vi "rszvl_core_global.vi"() -> ()   [LabVIEW 2014] (continued)
"*WAI"=FALSE}, "Check Status Callback"=""}, {"Level"=2, "Descriptive Name"="File Decimal Separator", "Class Only"=FALSE, "Data Type"=0, "Access"=2, "Identifier"="RSZVL_ATTR_FILE_DEC_SEPARATOR", "Range Table"="rszvl_rngFileDecSeparator", "Command"="FORM:DEXP:DSEP", "Read Callback"="", "Write Callback"="", "Range Callback"="", "Check Callback"="", "Rngtable Callback"="", "Coerce Callback"="", "User Callback"="", "Supported Models"="", "Instrument Options"="", "Repeated Capabilities"="", "Restricted Repeated Capabilities"="", "Help"="This attribute defines which decimal separator (decimal point or comma) is to be used for outputting measurement data to the file in ASCII format.\n\nAvailable Repeated Capabilities:\nNone\n\nRemote-control command(s):\nFORMat:DEXPort:DSEParator POINt|COMMa", "Flags"={"OPC Wait"=FALSE, "Dont check status"=FALSE, "*WAI"=FALSE}, "Check Status Callback"=""}, {"Level"=2, "Descriptive Name"="Manager", "Class Only"=TRUE, "Data Type"=0, "Access"=0, "Identifier"="", "Range Table"="", "Command"="", "Read Callback"="", "Write Callback"="", "Range Callback"="", "Check Callback"="", "Rngtable Callback"="", "Coerce Callback"="", "User Callback"="", "Supported Models"="", "Instrument Options"="", "Repeated Capabilities"="", "Restricted Repeated Capabilities"="", "Help"="File management attributes.\n\n(1) File Manager Edit Path:\nThis attribute changes the current directory.\nIn addition to the path name, the indication of the directory may contain the drive name. The path name complies with the DOS conventions.\n\n(2) File Manager Delete:\n\n\n(3) File Manager Make Directory:\nThis attribute creates a new directory. The file name includes indication of the path and may also include the drive name. The path name complies with DOS conventions.\n\n(4) File Manager Edit Path Device:\nThis attribute changes to the drive indicated. The drive may be the internal hard disk D: or the floppy disk drive A:.\n\n(5) File Manager Delete Directory:\nThis attribute deletes the indicated directory. The directory name includes indication of the path and may also include the drive name. The path name complies with DOS conventions.", "Flags"={"OPC Wait"=FALSE, "Dont check status"=FALSE, "*WAI"=FALSE}, "Check Status Callback"=""}, {"Level"=3, "Descriptive Name"="File Manager Edit Path", "Class Only"=FALSE, "Data Type"=2, "Access"=2, "Identifier"="RSZVL_ATTR_FILE_MANAGER_EDIT_PATH", "Range Table"="", "Command"="MMEM:CDIR", "Read Callback"="rszvl_quotedString_ReadCallback.vi", "Write Callback"="rszvl_quotedString_WriteCallback.vi", "Range Callback"="", "Check Callback"="", "Rngtable Callback"="", "Coerce Callback"="", "User Callback"="", "Supported Models"="", "Instrument Options"="", "Repeated Capabilities"="", "Restricted Repeated Capabilities"="", "Help"="This attribute changes the current directory.\nIn addition to the path name, the indication of the directory may contain the drive name. The path name complies with the DOS conventions.\n\nAvailable Repeated Capabilities:\nNone\n\nRemote-control command(s):\nMMEMory:CDIRectory", "Flags"={"OPC Wait"=FALSE, "Dont check status"=FALSE, "*WAI"=FALSE}, "Check Status Callback"=""}, {"Level"=3, "Descriptive Name"="File Manager Delete", "Class Only"=FALSE, "Data Type"=2, "Access"=1, "Identifier"="RSZVL_ATTR_FILE_MANAGER_DELETE", "Range Table"="", "Command"="MMEM:DEL", "Read Callback"="", "Write Callback"="", "Range Callback"="", "Check Callback"="", "Rngtable Callback"="", "Coerce Callback"="", "User Callback"="", "Supported Models"="", "Instrument Options"="", "Repeated Capabilities"="", "Restricted Repeated Capabilities"="", "Help"="\n\nAvailable Repeated Capabilities:\nNone\n\nRemote-control command(s):\nMMEMory:DELete", "Flags"={"OPC Wait"=FALSE, "Dont check status"=FALSE, "*WAI"=FALSE}, "Check Status Callback"=""}, {"Level"=3, "Descriptive Name"="File Manager Make Directory", "Class Only"=FALSE, "Data Type"=2, "Access"=2, "Identifier"="RSZVL_ATTR_FILE_MANAGER_MAKE_DIR", "Range Table"="", "Command"="MMEM:MDIR", "Read Callback"="", "Write Callback"="", "Range Callback"="", "Check Callback"="", "Rngtable Callback"="", "Coerce Callback"="", "User Callback"="", "Supported Models"="", "Instrument Options"="", "Repeated Capabilities"="", "Restricted Repeated Capabilities"="", "Help"="This attribute creates a new directory. The file name includes indication of the path and may also include the drive name. The path name complies with DOS conventions.\n\nAvailable Repeated Capabilities:\nNone\n\nRemote-control command(s):\nMMEMory:MDIRectory", "Flags"={"OPC Wait"=FALSE, "Dont check status"=FALSE, "*WAI"=FALSE}, "Check Status Callback"=""}, {"Level"=3, "Descriptive Name"="File Manager Edit Path Device", "Class Only"=FALSE, "Data Type"=2, "Access"=2, "Identifier"="RSZVL_ATTR_FILE_MANAGER_EDIT_PATH_DEVICE", "Range Table"="", "Command"="MMEM:MSIS", "Read Callback"="rszvl_quotedString_ReadCallback.vi", "Write Callback"="rszvl_quotedString_WriteCallback.vi", "Range Callback"="", "Check Callback"="", "Rngtable Callback"="", "Coerce Callback"="", "User Callback"="", "Supported Models"="", "Instrument Options"="", "Repeated Capabilities"="", "Restricted Repeated Capabilities"="", "Help"="This attribute changes to the drive indicated. The drive may be the internal hard disk D: or the floppy disk drive A:.\n\nAvailable Repeated Capabilities:\nNone\n\nRemote-control command(s):\nMMEMory:MSIS", "Flags"={"OPC Wait"=FALSE, "Dont check status"=FALSE, "*WAI"=FALSE}, "Check Status Callback"=""}, {"Level"=3, "Descriptive Name"="File Manager Delete Directory", "Class Only"=FALSE, "Data Type"=2, "Access"=2, "Identifier"="RSZVL_ATTR_FILE_MANAGER_DELETE_DIR", "Range Table"="", "Command"="MMEM:RDIR", "Read Callback"="", "Write Callback"="", "Range Callback"="", "Check Callback"="", "Rngtable Callback"="", "Coerce Callback"="", "User Callback"="", "Supported Models"="", "Instrument Options"="", "Repeated Capabilities"="", "Restricted Repeated Capabilities"="", "Help"="This attribute deletes the indicated directory. The directory name includes indication of the path and may also include the drive name. The path name complies with DOS conventions.\n\nAvailable Repeated Capabilities:\nNone\n\nRemote-control command(s):\nMMEMory:RDIRectory", "Flags"={"OPC Wait"=FALSE, "Dont check status"=FALSE, "*WAI"=FALSE}, "Check Status Callback"=""}, {"Level"=2, "Descriptive Name"="Save Recall", "Class Only"=TRUE, "Data Type"=0, "Access"=0, "Identifier"="", "Range Table"="", "Command"="", "Read Callback"="", "Write Callback"="", "Range Callback"="", "Check Callback"="", "Rngtable Callback"="", "Coerce Callback"="", "User Callback"="", "Supported Models"="", "Instrument Options"="", "Repeated Capabilities"="", "Restricted Repeated Capabilities"="", "Help"="Configuration of stored setups.\n\n(1) File Items to Save Recall Select Source Cal Data:\nThis attribute adds the tracking generator calibration data to the list of device settings to be stored/loaded.\n\n(2) File Items to Save Recall Select All Transducers:\nThis attribute includes all transducer factors and sets in the list of data subsets of a device setting to be stored/loaded.\n\n(3) File Items to Save Recall Select HW Settings:\nThis attribute includes the hardware settings in the list of data subsets of a device setting to be stored/loaded. The hardware settings include:\n- current configuration of general device parameters (general setup)\n- current setting of the measurement hardware including markers\n- activated limit lines:\nA data set may include 8 limit lines at maximum. This number includes the activated limit lines and, if available, the de-activated limit lines last used. Therefore the combination of the non-activated restored limit lines depends on the sequence of use with the command MMEM:LOAD.\n- user-defined color setting\n- configuration for the hardcopy output\n- Tracking generator settings (only in conjunction with option External Generator Control B10)\n- Correction data for source calibration (only in conjunction with option External Generator Control B10)\n\n(4) File Items to Save Recall Select Trace:\nThis attribute adds the active traces to the list of data subsets of a save/recall device setting. Active traces are all traces whose state is not blank.\n\n(5) File Items to Save Recall Select Lines:\nThis attribute adds all limit lines (activated and de-activated) to the list of device settings to be\nstored/loaded.\n\n(6) File Items to Save Recall All:\nThis command includes all data subsets in the list device settings to be stored/loaded.\n\n(7) File Items to Save Recall None:\nThis attribute deletes all data subsets from the list of device settings to be stored/loaded.\n\n(8) File Items to Save Recall Default:\nThis attribute sets the default list of device settings to be stored/loaded.The latter includes:\n- current configuration of general device parameters (general setup)\n- current setting of the measurement hardware including markers\n- activated limit lines\n- user-defined color setting\n- configuration for the hardcopy output\n- Tracking generator settings (only in conjunction with option External Generator Control B10)\n- Correction data for source calibration (only in conjunction with option External Generator Control B10)\nTrace data and non-used limit lines are not included.", "Flags"={"OPC Wait"=FALSE, "Dont check status"=FALSE, "*WAI"=FALSE}, "Check Status Callback"=""}, {"Level"=3, "Descriptive Name"="File Items to Save Recall Select Source Cal Data", "Class Only"=FALSE, "Data Type"=3, "Access"=2, "Identifier"="RSZVL_ATTR_FILE_ITEMS_SAVE_RECAL_SEL_SOURCE_CAL_DATA", "Range Table"="", "Command"="MMEM:SEL:SCD", "Read Callback"="", "Write Callback"="", "Range Callback"="", "Check Callback"="", "Rngtable Callback"="", "Coerce Callback"="", "User Callback"="", "Supported Models"="", "Instrument Options"="", "Repeated Capabilities"="", "Restricted Repeated Capabilities"="", "Help"="This attribute adds the tracking generator calibration data to the list of device settings to be stored/loaded.\n\nAvailable Repeated Capabilities:\nNone\n\nRemote-control command(s):\nMMEMory:SELect[:ITEM]:SCData ON | OFF", "Flags"={"OPC Wait"=FALSE, "Dont check status"=FALSE, "*WAI"=FALSE}, "Check Status Callback"=""}, {"Level"=3, "Descriptive Name"="File Items to Save Recall Select All Transducers", "Class Only"=FALSE, "Data Type"=3, "Access"=2, "Identifier"="RSZVL_ATTR_FILE_ITEMS_SAVE_RECAL_SEL_TRAN", "Range Table"="", "Command"="MMEM:SEL:TRAN:ALL", "Read Callback"="", "Write Callback"="", "Range Callback"="", "Check Callback"="", "Rngtable Callback"="", "Coerce Callback"="", "User Callback"="", "Supported Models"="", "Instrument Options"="", "Repeated Capabilities"="", "Restricted Repeated Capabilities"="", "Help"="This attribute includes all transducer factors and sets in the list of data subsets of a device setting to be stored/loaded.\n\nAvailable Repeated Capabilities:\nNone\n\nRemote-control command(s):\nMMEMory:SELect[:ITEM]:TRANsducer:ALL ON | OFF", "Flags"={"OPC Wait"=FALSE, "Dont check status"=FALSE, "*WAI"=FALSE}, "Check Status Callback"=""}, {"Level"=3, "Descriptive Name"="File Items to Save Recall Select HW Settings", "Class Only"=FALSE, "Data Type"=3, "Access"=2, "Identifier"="RSZVL_ATTR_FILE_ITEMS_SAVE_RECAL_SEL_HWSETTINGS", "Range Table"="", "Command"="MMEM:SEL:HWS", "Read Callback"="", "Write Callback"="", "Range Callback"="", "Check Callback"="", "Rngtable Callback"="", "Coerce Callback"="", "User Callback"="", "Supported Models"="", "Instrument Options"="", "Repeated Capabilities"="", "Restricted Repeated Capabilities"="", "Help"="This attribute includes the hardware settings in the list of data subsets of a device setting to be stored/loaded. The hardware settings include:\n- current configuration of general device parameters (general setup)\n- current setting of the measurement hardware including markers\n- activated limit lines:\nA data set may include 8 limit lines at maximum. This number includes the activated limit lines and, if available, the de-activated limit lines last used. Therefore the combination of the non-activated restored limit lines depends on the sequence of use with the command MMEM:LOAD.\n- user-defined color setting\n- configuration for the hardcopy output\n- Tracking generator settings (only in conjunction with option External Generator Control B10)\n- Correction data for source calibration (only in conjunction with option External Generator Control B10)\n\nAvailable Repeated Capabilities:\nNone\n\nRemote-control command(s):\nMMEMory:SELect[:ITEM]:HWSettings ON|OFF", "Flags"={"OPC Wait"=FALSE, "Dont check status"=FALSE, "*WAI"=FALSE}, "Check Status Callback"=""}, {"Level"=3, "Descriptive Name"="File Items to Save Recall Select Trace", "Class Only"=FALSE, "Data Type"=3, "Access"=2, "Identifier"="RSZVL_ATTR_FILE_ITEMS_SAVE_RECAL_SEL_TRAC", "Range Table"="", "Command"="MMEM:SEL:TRAC", "Read Callback"="", "Write Callback"="", "Range Callback"="", "Check Callback"="", "Rngtable Callback"="", "Coerce Callback"="", "User Callback"="", "Supported Models"="", "Instrument Options"="", "Repeated Capabilities"="", "Restricted Repeated Capabilities"="", "Help"="This attribute adds the active traces to the list of data subsets of a save/recall device setting. Active traces are all traces whose state is not blank.\n\nAvailable Repeated Capabilities:\nNone\n\nRemote-control command(s):\nMMEMory:SELect[:ITEM]:TRACe[:ACTive] ON|OFF", "Flags"={"OPC Wait"=FALSE, "Dont check status"=FALSE, "*WAI"=FALSE}, "Check Status Callback"=""}, {"Level"=3, "Descriptive Name"="File Items to Save Recall Select Lines", "Class Only"=FALSE, "Data Type"=3, "Access"=2, "Identifier"="RSZVL_ATTR_FILE_ITEMS_SAVE_RECAL_SEL_LINE", "Range Table"="", "Command"="MMEM:SEL:LIN:ALL", "Read Callback"="", "Write Callback"="", "Range Callback"="", "Check Callback"="", "Rngtable Callback"="", "Coerce Callback"="", "User Callback"="", "Supported Models"="", "Instrument Options"="", "Repeated Capabilities"="", "Restricted Repeated Capabilities"="", "Help"="This attribute adds all limit lines (activated and de-activated) to the list of device settings to be\nstored/loaded.\n\nAvailable Repeated Capabilities:\nNone\n\nRemote-control command(s):\nMMEMory:SELect[:ITEM]:LINes:ALL ON|OFF", "Flags"={"OPC Wait"=FALSE, "Dont check status"=FALSE, "*WAI"=FALSE}, "Check Status Callback"=""}, {"Level"=3, "Descriptive Name"="File Items to Save Recall All", "Class Only"=FALSE, "Data Type"=4, "Access"=1, "Identifier"="RSZVL_ATTR_FILE_ITEMS_SAVE_RECAL_ALL", "Range Table"="", "Command"="MMEM:SEL:ALL", "Read Callback"="", "Write Callback"="", "Range Callback"="", "Check Callback"="", "Rngtable Callback"="", "Coerce Callback"="", "User Callback"="", "Supported Models"="", "Instrument Options"="", "Repeated Capabilities"="", "Restricted Repeated Capabilities"="", "Help"="This command includes all data subsets in the list device settings to be stored/loaded.\n\nAvailable Repeated Capabilities:\nNone\n\nRemote-control command(s):\nMMEMory:SELect[:ITEM]:ALL", "Flags"={"OPC Wait"=FALSE, "Dont check status"=FALSE, "*WAI"=FALSE}, "Check Status Callback"=""}, {"Level"=3, "Descriptive Name"="File Items to Save Recall None", "Class Only"=FALSE, "Data Type"=4, "Access"=1, "Identifier"="RSZVL_ATTR_FILE_ITEMS_SAVE_RECAL_NONE", "Range Table"="", "Command"="MMEM:SEL:NONE", "Read Callback"="", "Write Callback"="", "Range Callback"="", "Check Callback"="", "Rngtable Callback"="", "Coerce Callback"="", "User Callback"="", "Supported Models"="", "Instrument Options"="", "Repeated Capabilities"="", "Restricted Repeated Capabilities"="", "Help"="This attribute deletes all data subsets from the list of device settings to be stored/loaded.\n\nAvailable Repeated Capabilities:\nNone\n\nRemote-control command(s):\nMMEMory:SELect[:ITEM]:NONE", "Flags"={"OPC Wait"=FALSE, "Dont check status"=FALSE, "*WAI"=FALSE}, "Check Status Callback"=""}, {"Level"=3, "Descriptive Name"="File Items to Save Recall Default", "Class Only"=FALSE, "Data Type"=4, "Access"=1, "Identifier"="RSZVL_ATTR_FILE_ITEMS_SAVE_RECAL_DEFAULT", "Range Table"="", "Command"="MMEM:SEL:DEF", "Read Callback"="", "Write Callback"="", "Range Callback"="", "Check Callback"="", "Rngtable Callback"="", "Coerce Callback"="", "User Callback"="", "Supported Models"="", "Instrument Options"="", "Repeated Capabilities"="", "Restricted Repeated Capabilities"="", "Help"="This attribute sets the default list of device settings to be stored/loaded.The latter includes:\n- current configuration of general device parameters (general setup)\n- current setting of the measurement hardware including markers\n- activated limit lines\n- user-defined color setting\n- configuration for the hardcopy output\n- Tracking generator settings (only in conjunction with option External Generator Control B10)\n- Correction data for source calibration (only in conjunction with option External Generator Control B10)\nTrace data and non-used limit lines are not included.\n\nAvailable Repeated Capabilities:\nNone\n\nRemote-control command(s):\nMMEMory:SELect[:ITEM]:DEFault", "Flags"={"OPC Wait"=FALSE, "Dont check status"=FALSE, "*WAI"=FALSE}, "Check Status Callback"=""}, {"Level"=1, "Descriptive Name"="Hard Copy", "Class Only"=TRUE, "Data Type"=0, "Access"=0, "Identifier"="", "Range Table"="", "Command"="", "Read Callback"="", "Write Callback"="", "Range Callback"="", "Check Callback"="", "Rngtable Callback"="", "Coerce Callback"="", "User Callback"="", "Supported Models"="", "Instrument Options"="", "Repeated Capabilities"="", "Restricted Repeated Capabilities"="", "Help"="(1) Hcopy Abort:\nThis attribute aborts a running hardcopy output.\n\n(2) Hcopy Color Default:\nThis attribute resets the colors for a hardcopy to the selected default settings. DEFault1(SCREEN COLORS, but background white), DEFault2 (OPTIMIZED COLOR SET) and DEFault3 (USER DEFINED). The numeric suffix in CMAP is not significant.\n\n(3) Hcopy Color:\nThis attribute selects between color and monochrome hardcopy of the screen.\n\n(4) Hcopy Print:\nThis attribute starts a hardcopy output. The numeric suffix selects which printer configuration (1 or 2) is to be used for the hardcopy output. If there is no suffix, configuration 1 is automatically selected.\n\n(5) Hcopy Print Next:\nThis attribute starts a hardcopy output. If the output is printed to a file (see HCOPy:DESTination<1|2>), the file name used in the last saving process is automatically counted up to the next unused name.\n\n(6) Hcopy Device Destination:\nThis attribute selects the printer output medium (Disk, Printer or Clipboard) associated with configuration 1 or 2.\n\n(7) Hcopy Color Predefined:\nThis attribute defines the color table in USER DEFINED COLORS using predefined color values. To each numeric suffix of CMAP is assigned one or several picture elements which can be modified by varying the corresponding color setting.\n\n(8) Hcopy Device Language Output Format:\nThis attribute determines the data format of the printout. More info in manual.\n\n(9) Hcopy Print Screen:\nThis attribute selects the complete screen to be output.\n\n(10) Hcopy Comment Screen:\nThis attribute defines the comment text for printout, with a maximum of 100 characters; line feed by means of character @).\n\n(11) Hcopy Print Trace:\nThis attribute selects the output of the currently displayed trace.\n\n(12) Hcopy Device Orientation:\n\n\n(13) Hcopy File Name:\nThis attribute defines a destination file for the printout started with the command HCOPy:IMMediate. In this case the printer output must be routed to destination FILE using the attribute RSZVL_ATTR_HCOPY_DEVICE_DESTINATION with MMEM\nThe file name includes indication of the path and may also include the drive name. The file name and path information comply with DOS conventions.\n\n(14) Hardcopy Select Printer:\nThis attribute selects one of the printers configured under Windows NT including the associated output destination.\n\nThe specified printer name must be a string as returned by the commands\nSYSTem:COMMunicate :PRINter:ENUMerate:FIRSt? or\nSYSTem:COMMunicate :PRINter:ENUMerate:NEXT?\n\n(15) Hardcopy Get Next Printer:\nThis attribute queries the name of the next printer installed under Windows NT.\nThe names of other printers can then be queried with NEXT?. After all available printer names have been output, an empty string enclosed by quotation marks is output for the next query. Further queries are answered by a Query Error.\n\n(16) Hardcopy Get First Printer:\nThis attribute queries the name of the first printer (in the list of printers) available under Windows NT.", "Flags"={"OPC Wait"=FALSE, "Dont check status"=FALSE, "*WAI"=FALSE}, "Check Status Callback"=""}, {"Level"=2, "Descriptive Name"="Hcopy Abort", "Class Only"=FALSE, "Data Type"=4, "Access"=1, "Identifier"="RSZVL_ATTR_HCOPY_ABORT", "Range Table"="", "Command"="HCOP:ABOR", "Read Callback"="", "Write Callback"="", "Range Callback"="", "Check Callback"="", "Rngtable Callback"="", "Coerce Callback"="", "User Callback"="", "Supported Models"="", "Instrument Options"="", "Repeated Capabilities"="", "Restricted Repeated Capabilities"="", "Help"="This attribute aborts a running hardcopy output.\n\nAvailable Repeated Capabilities:\nNone\n\nRemote-control command(s):\nHCOPy:ABORt", "Flags"={"OPC Wait"=FALSE, "Dont check status"=FALSE, "*WAI"=FALSE}, "Check Status Callback"=""}, {"Level"=2, "Descriptive Name"="Hcopy Color Default", "Class Only"=FALSE, "Data Type"=4, "Access"=1, "Identifier"="RSZVL_ATTR_HCOPY_COLOR_DEF", "Range Table"="", "Command"="HCOP:CMAP:DEF{Default}", "Read Callback"="", "Write Callback"="", "Range Callback"="", "Check Callback"="", "Rngtable Callback"="", "Coerce Callback"="", "User Callback"="", "Supported Models"="", "Instrument Options"="", "Repeated Capabilities"="", "Restricted Repeated Capabilities"="", "Help"="This attribute resets the colors for a hardcopy to the selected default settings. DEFault1(SCREEN COLORS, but background white), DEFault2 (OPTIMIZED COLOR SET) and DEFault3 (USER DEFINED). The numeric suffix in CMAP is not significant.\n\nAvailable Repeated Capabilities:\nDefault: DEF1,DEF2,DEF3\r\n\nRemote-control command(s):\nHCOPy:CMAP<1 to 27>:DEFault1|2|3", "Flags"={"OPC Wait"=FALSE, "Dont check status"=FALSE, "*WAI"=FALSE}, "Check Status Callback"=""}, {"Level"=2, "Descriptive Name"="Hcopy Color", "Class Only"=FALSE, "Data Type"=3, "Access"=2, "Identifier"="RSZVL_ATTR_HCOPY_COLOR", "Range Table"="", "Command"="HCOP:DEV:COL", "Read Callback"="", "Write Callback"="", "Range Callback"="", "Check Callback"="", "Rngtable Callback"="", "Coerce Callback"="", "User Callback"="", "Supported Models"="", "Instrument Options"="", "Repeated Capabilities"="", "Restricted Repeated Capabilities"="", "Help"="This attribute selects between color and monochrome hardcopy of the screen.\n\nAvailable Repeated Capabilities:\nNone\n\nRemote-control command(s):\nHCOPy:DEVice:COLor ON|OFF", "Flags"={"OPC Wait"=FALSE, "Dont check status"=FALSE, "*WAI"=FALSE}, "Check Status Callback"=""}, {"Level"=2, "Descriptive Name"="Hcopy Print", "Class Only"=FALSE, "Data Type"=4, "Access"=1, "Identifier"="RSZVL_ATTR_HCOPY_PRINT", "Range Table"="", "Command"="HCOP:IMM{Destination}", "Read Callback"="", "Write Callback"="", "Range Callback"="", "Check Callback"="", "Rngtable Callback"="", "Coerce Callback"="", "User Callback"="", "Supported Models"="", "Instrument Options"="", "Repeated Capabilities"="", "Restricted Repeated Capabilities"="", "Help"="This attribute starts a hardcopy output. The numeric suffix selects which printer configuration (1 or 2) is to be used for the hardcopy output. If there is no suffix, configuration 1 is automatically selected.\n\nAvailable Repeated Capabilities:\nDestination: DE1,DE2\r\n\nRemote-control command(s):\nHCOPy[:IMMediate<1|2>]", "Flags"={"OPC Wait"=FALSE, "Dont check status"=FALSE, "*WAI"=FALSE}, "Check Status Callback"=""}, {"Level"=2, "Descriptive Name"="Hcopy Print Next", "Class Only"=FALSE, "Data Type"=4, "Access"=1, "Identifier"="RSZVL_ATTR_HCOPY_PRINT_NEXT", "Range Table"="", "Command"="HCOP:IMM{Destination}:NEXT", "Read Callback"="", "Write Callback"="", "Range Callback"="", "Check Callback"="", "Rngtable Callback"="", "Coerce Callback"="", "User Callback"="", "Supported Models"="", "Instrument Options"="", "Repeated Capabilities"="", "Restricted Repeated Capabilities"="", "Help"="This attribute starts a hardcopy output. If the output is printed to a file (see HCOPy:DESTination<1|2>), the file name used in the last saving process is automatically counted up to the next unused name.\n\nAvailable Repeated Capabilities:\nDestination: DE1,DE2\r\n\nRemote-control command(s):\nHCOPy[:IMMediate<config>]:NEXT", "Flags"={"OPC Wait"=FALSE, "Dont check status"=FALSE, "*WAI"=FALSE}, "Check Status Callback"=""}, {"Level"=2, "Descriptive Name"="Hcopy Device Destination", "Class Only"=FALSE, "Data Type"=0, "Access"=2, "Identifier"="RSZVL_ATTR_HCOPY_DEVICE_DESTINATION", "Range Table"="rszvl_rngHcopyDevice", "Command"="HCOP:DEST{Destination}", "Read Callback"="", "Write Callback"="", "Range Callback"="", "Check Callback"="", "Rngtable Callback"="", "Coerce Callback"="", "User Callback"="", "Supported Models"="", "Instrument Options"="", "Repeated Capabilities"="", "Restricted Repeated Capabilities"="", "Help"="This attribute selects the printer output medium (Disk, Printer or Clipboard) associated with configuration 1 or 2.\n\nAvailable Repeated Capabilities:\nDestination: DE1,DE2\r\n\nRemote-control command(s):\nHCOPy:DESTination<1|2>", "Flags"={"OPC Wait"=FALSE, "Dont check status"=FALSE, "*WAI"=FALSE}, "Check Status Callback"=""}, {"Level"=2, "Descriptive Name"="Hcopy Color Predefined", "Class Only"=FALSE, "Data Type"=0, "Access"=1, "Identifier"="RSZVL_ATTR_HCOPY_COLOR_PREDEFINED", "Range Table"="rszvl_rngDISPConfPreDefColour", "Command"="HCOP:CMAP{CMAP}:PDEF", "Read Callback"="", "Write Callback"="", "Range Callback"="", "Check Callback"="", "Rngtable Callback"="", "Coerce Callback"="", "User Callback"="", "Supported Models"="", "Instrument Options"="", "Repeated Capabilities"="", "Restricted Repeated Capabilities"="", "Help"="This attribute defines the color table in USER DEFINED COLORS using predefined color values. To each numeric suffix of CMAP is assigned one or several picture elements which can be modified by varying the corresponding color setting.\n\nAvailable Repeated Capabilities:\nCMAP: CM1,CM2,CM3,CM4,CM5,CM6,CM7,CM8,CM9,CM10,CM11,CM12,CM13,CM14,CM15,CM16,CM17,CM18,CM19,CM20,CM21,CM22,CM23,CM24,CM25,CM26,CM27\r\n\nRemote-control command(s):\nHCOPy:CMAP<1 to 26>:PDEFined BLACk | BLUE | BROWn | GREen | CYAN | RED | MAGenta | YELLow | WHITe | DGRAy | LGRAy | LBLUe | LGREen | LCYan | LRED | LMAGenta", "Flags"={"OPC Wait"=FALSE, "Dont check status"=FALSE, "*WAI"=FALSE}, "Check Status Callback"=""}, {"Level"=2, "Descriptive Name"="Hcopy Device Language Output Format", "Class Only"=FALSE, "Data Type"=0, "Access"=2, "Identifier"="RSZVL_ATTR_HCOPY_DEVICE_LANG_OUT_FORM", "Range Table"="rszvl_rngHcopyDeviceLang", "Command"="HCOP:DEV:LANG", "Read Callback"="", "Write Callback"="", "Range Callback"="", "Check Callback"="", "Rngtable Callback"="", "Coerce Callback"="", "User Callback"="", "Supported Models"="", "Instrument Options"="", "Repeated Capabilities"="", "Restricted Repeated Capabilities"="", "Help"="This attribute determines the data format of the printout. More info in manual.\n\nAvailable Repeated Capabilities:\nNone\n\nRemote-control command(s):\nHCOPy:DEVice:LANGuage<1|2> GDI | WMF | EWMF | BMP", "Flags"={"OPC Wait"=FALSE, "Dont check status"=FALSE, "*WAI"=FALSE}, "Check Status Callback"=""}, {"Level"=2, "Descriptive Name"="Hcopy Print Screen", "Class Only"=FALSE, "Data Type"=4, "Access"=1, "Identifier"="RSZVL_ATTR_HCOPY_PRINT_SCREEN", "Range Table"="", "Command"="HCOP:ITEM:ALL", "Read Callback"="", "Write Callback"="", "Range Callback"="", "Check Callback"="", "Rngtable Callback"="", "Coerce Callback"="", "User Callback"="", "Supported Models"="", "Instrument Options"="", "Repeated Capabilities"="", "Restricted Repeated Capabilities"="", "Help"="This attribute selects the complete screen to be output.\n\nAvailable Repeated Capabilities:\nNone\n\nRemote-control command(s):\nHCOPy:ITEM:ALL", "Flags"={"OPC Wait"=FALSE, "Dont check status"=FALSE, "*WAI"=FALSE}, "Check Status Callback"=""}, {"Level"=2, "Descriptive Name"="Hcopy Comment Screen", "Class Only"=FALSE, "Data Type"=2, "Access"=2, "Identifier"="RSZVL_ATTR_HCOPY_COMM_SCR", "Range Table"="", "Command"="HCOP:ITEM:WIND:TEXT", "Read Callback"="rszvl_quotedString_ReadCallback.vi", "Write Callback"="rszvl_quotedString_WriteCallback.vi", "Range Callback"="", "Check Callback"="", "Rngtable Callback"="", "Coerce Callback"="", "User Callback"="", "Supported Models"="", "Instrument Options"="", "Repeated Capabilities"="", "Restricted Repeated Capabilities"="", "Help"="This attribute defines the comment text for printout, with a maximum of 100 characters; line feed by means of character @).\n\nAvailable Repeated Capabilities:\nNone\n\nRemote-control command(s):\nHCOPy:ITEM:WINDow<1|2>:TEXT", "Flags"={"OPC Wait"=FALSE, "Dont check status"=FALSE, "*WAI"=FALSE}, "Check Status Callback"=""}, {"Level"=2, "Descriptive Name"="Hcopy Print Trace", "Class Only"=FALSE, "Data Type"=3, "Access"=2, "Identifier"="RSZVL_ATTR_HCOPY_PRINT_TRACE", "Range Table"="", "Command"="HCOP:ITEM:WIND:TRAC:STAT", "Read Callback"="", "Write Callback"="", "Range Callback"="", "Check Callback"="", "Rngtable Callback"="", "Coerce Callback"="", "User Callback"="", "Supported Models"="", "Instrument Options"="", "Repeated Capabilities"="", "Restricted Repeated Capabilities"="", "Help"="This attribute selects the output of the currently displayed trace.\n\nAvailable Repeated Capabilities:\nNone\n\nRemote-control command(s):\nHCOPy:ITEM:WINDow<1|2>:TRACe:STATe ON | OFF", "Flags"={"OPC Wait"=FALSE, "Dont check status"=FALSE, "*WAI"=FALSE}, "Check Status Callback"=""}, {"Level"=2, "Descriptive Name"="Hcopy Device Orientation", "Class Only"=FALSE, "Data Type"=0, "Access"=2, "Identifier"="RSZVL_ATTR_HCOPY_DEVICE_ORIENTATION", "Range Table"="rszvl_rngHcopyDeviceOrient", "Command"="HCOP:PAGE:ORI{Destination}", "Read Callback"="", "Write Callback"="", "Range Callback"="", "Check Callback"="", "Rngtable Callback"="", "Coerce Callback"="", "User Callback"="", "Supported Models"="", "Instrument Options"="", "Repeated Capabilities"="", "Restricted Repeated Capabilities"="", "Help"="\n\nAvailable Repeated Capabilities:\nDestination: DE1,DE2\r\n\nRemote-control command(s):\nHCOPy:PAGE:ORIentation<1|2> LANDscape | PORTrait", "Flags"={"OPC Wait"=FALSE, "Dont check status"=FALSE, "*WAI"=FALSE}, "Check Status Callback"=""}, {"Level"=2, "Descriptive Name"="Hcopy File Name", "Class Only"=FALSE, "Data Type"=2, "Access"=2, "Identifier"="RSZVL_ATTR_HCOPY_FILE_NAME", "Range Table"="", "Command"="MMEM:NAME", "Read Callback"="rszvl_quotedString_ReadCallback.vi", "Write Callback"="rszvl_quotedString_WriteCallback.vi", "Range Callback"="", "Check Callback"="", "Rngtable Callback"="", "Coerce Callback"="", "User Callback"="", "Supported Models"="", "Instrument Options"="", "Repeated Capabilities"="", "Restricted Repeated Capabilities"="", "Help"="This attribute defines a destination file for the printout started with the command HCOPy:IMMediate. In this case the printer output must be routed to destination FILE using the attribute RSZVL_ATTR_HCOPY_DEVICE_DESTINATION with MMEM\nThe file name includes indication of the path and may also include the drive name. The file name and path information comply with DOS conventions.\n\nAvailable Repeated Capabilities:\nNone\n\nRemote-control command(s):\nMMEMory:NAME", "Flags"={"OPC Wait"=FALSE, "Dont check status"=FALSE, "*WAI"=FALSE}, "Check Status Callback"=""}, {"Level"=2, "Descriptive Name"="Hardcopy Select Printer", "Class Only"=FALSE, "Data Type"=2, "Access"=2, "Identifier"="RSZVL_ATTR_HCOPY_PRINTER", "Range Table"="", "Command"="SYST:COMM:PRIN:SEL{Destination}", "Read Callback"="rszvl_quotedString_ReadCallback.vi", "Write Callback"="rszvl_quotedString_WriteCallback.vi", "Range Callback"="", "Check Callback"="", "Rngtable Callback"="", "Coerce Callback"="", "User Callback"="", "Supported Models"="", "Instrument Options"="", "Repeated Capabilities"="", "Restricted Repeated Capabilities"="", "Help"="This attribute selects one of the printers configured under Windows NT including the associated output destination.\n\nThe specified printer name must be a string as returned by the commands\nSYSTem:COMMunicate :PRINter:ENUMerate:FIRSt? or\nSYSTem:COMMunicate :PRINter:ENUMerate:NEXT?\n\nAvailable Repeated Capabilities:\nDestination: DE1,DE2\r\n\nRemote-control command(s):\nSYSTem:COMMunicate:PRINter:SELect <1|2> <printer_name>", "Flags"={"OPC Wait"=FALSE, "Dont check status"=FALSE, "*WAI"=FALSE}, "Check Status Callback"=""}, {"Level"=2, "Descriptive Name"="Hardcopy Get Next Printer", "Class Only"=FALSE, "Data Type"=2, "Access"=0, "Identifier"="RSZVL_ATTR_HCOPY_PRINTER_NEXT", "Range Table"="", "Command"="SYST:COMM:PRIN:ENUM:NEXT?", "Read Callback"="", "Write Callback"="", "Range Callback"="", "Check Callback"="", "Rngtable Callback"="", "Coerce Callback"="", "User Callback"="", "Supported Models"="", "Instrument Options"="", "Repeated Capabilities"="", "Restricted Repeated Capabilities"="", "Help"="This attribute queries the name of the next printer installed under Windows NT.\nThe names of other printers can then be queried with NEXT?. After all available printer names have been output, an empty string enclosed by quotation marks is output for the next query. Further queries are answered by a Query Error.\n\nAvailable Repeated Capabilities:\nNone\n\nRemote-control command(s):\nSYSTem:COMMunicate:PRINter:ENUMerate:NEXT?", "Flags"={"OPC Wait"=FALSE, "Dont check status"=FALSE, "*WAI"=FALSE}, "Check Status Callback"=""}, {"Level"=2, "Descriptive Name"="Hardcopy Get First Printer", "Class Only"=FALSE, "Data Type"=2, "Access"=0, "Identifier"="RSZVL_ATTR_HCOPY_PRINTER_FIRST", "Range Table"="", "Command"="SYST:COMM:PRIN:ENUM:FIRS?", "Read Callback"="", "Write Callback"="", "Range Callback"="", "Check Callback"="", "Rngtable Callback"="", "Coerce Callback"="", "User Callback"="", "Supported Models"="", "Instrument Options"="", "Repeated Capabilities"="", "Restricted Repeated Capabilities"="", "Help"="This attribute queries the name of the first printer (in the list of printers) available under Windows NT.\n\nAvailable Repeated Capabilities:\nNone\n\nRemote-control command(s):\nSYSTem:COMMunicate:PRINter:ENUMerate:FIRSt?", "Flags"={"OPC Wait"=FALSE, "Dont check status"=FALSE, "*WAI"=FALSE}, "Check Status Callback"=""}, {"Level"=1, "Descriptive Name"="Reference Oscillator", "Class Only"=TRUE, "Data Type"=0, "Access"=0, "Identifier"="", "Range Table"="", "Command"="", "Read Callback"="", "Write Callback"="", "Range Callback"="", "Check Callback"="", "Rngtable Callback"="", "Coerce Callback"="", "User Callback"="", "Supported Models"="", "Instrument Options"="", "Repeated Capabilities"="", "Restricted Repeated Capabilities"="", "Help"="(1) Reference Oscillator Source:\nThis attribute selects the reference oscillator. If the external reference oscillator is selected, the reference signal must be connected to the rear panel of the instrument.", "Flags"={"OPC Wait"=FALSE, "Dont check status"=FALSE, "*WAI"=FALSE}, "Check Status Callback"=""}, {"Level"=2, "Descriptive Name"="Reference Oscillator Source", "Class Only"=FALSE, "Data Type"=0, "Access"=2, "Identifier"="RSZVL_ATTR_ROSC_SOURCE", "Range Table"="rszvl_rngSourceIntExt", "Command"="ROSC:SOUR", "Read Callback"="", "Write Callback"="", "Range Callback"="", "Check Callback"="", "Rngtable Callback"="", "Coerce Callback"="", "User Callback"="", "Supported Models"="", "Instrument Options"="", "Repeated Capabilities"="", "Restricted Repeated Capabilities"="", "Help"="This attribute selects the reference oscillator. If the external reference oscillator is selected, the reference signal must be connected to the rear panel of the instrument.\n\nAvailable Repeated Capabilities:\nNone\n\nRemote-control command(s):\n[SENSe<1|2>:]ROSCillator:SOURce INTernal | EXTernal", "Flags"={"OPC Wait"=FALSE, "Dont check status"=FALSE, "*WAI"=FALSE}, "Check Status Callback"=""}, {"Level"=1, "Descriptive Name"="System", "Class Only"=TRUE, "Data Type"=0, "Access"=0, "Identifier"="", "Range Table"="", "Command"="", "Read Callback"="", "Write Callback"="", "Range Callback"="", "Check Callback"="", "Rngtable Callback"="", "Coerce Callback"="", "User Callback"="", "Supported Models"="", "Instrument Options"="", "Repeated Capabilities"="", "Restricted Repeated Capabilities"="", "Help"="(1) System Error:\nThis attribute queries the earliest entry in the error queue, and deletes it after the readout.\n\n(2) System Error List:\nThis attribute command reads all system messages and returns a list of comma separated strings. Each\nstring corresponds to an entry in the table SYSTEM MESSAGES.\n\n(3) Clear Errors:\nThis attribute deletes all entries in the table SYSTEM MESSAGES.\n\n(4) System Preset:\nThis attribute initiates an instrument reset.\n\n(5) System Version:\nThis attribute queries the system version.\n\n(6) Speaker Volume:\nThis attribute sets the volume of the built-in loudspeaker for demodulated signals.", "Flags"={"OPC Wait"=FALSE, "Dont check status"=FALSE, "*WAI"=FALSE}, "Check Status Callback"=""}, {"Level"=2, "Descriptive Name"="System Error", "Class Only"=FALSE, "Data Type"=2, "Access"=0, "Identifier"="RSZVL_ATTR_SYST_ERR", "Range Table"="", "Command"="SYST:ERR?", "Read Callback"="", "Write Callback"="", "Range Callback"="", "Check Callback"="", "Rngtable Callback"="", "Coerce Callback"="", "User Callback"="", "Supported Models"="", "Instrument Options"="", "Repeated Capabilities"="", "Restricted Repeated Capabilities"="", "Help"="This attribute queries the earliest entry in the error queue, and deletes it after the readout.\n\nAvailable Repeated Capabilities:\nNone\n\nRemote-control command(s):\nSYSTem:ERRor?", "Flags"={"OPC Wait"=FALSE, "Dont check status"=FALSE, "*WAI"=FALSE}, "Check Status Callback"=""}, {"Level"=2, "Descriptive Name"="System Error List", "Class Only"=FALSE, "Data Type"=2, "Access"=0, "Identifier"="RSZVL_ATTR_SYST_ERR_LIST", "Range Table"="", "Command"="SYST:ERR:LIST?", "Read Callback"="", "Write Callback"="", "Range Callback"="", "Check Callback"="", "Rngtable Callback"="", "Coerce Callback"="", "User Callback"="", "Supported Models"="", "Instrument Options"="", "Repeated Capabilities"="", "Restricted Repeated Capabilities"="", "Help"="This attribute command reads all system messages and returns a list of comma separated strings. Each\nstring corresponds to an entry in the table SYSTEM MESSAGES.\n\nAvailable Repeated Capabilities:\nNone\n\nRemote-control command(s):\nSYSTem:ERRor:LIST?", "Flags"={"OPC Wait"=FALSE, "Dont check status"=FALSE, "*WAI"=FALSE}, "Check Status Callback"=""}, {"Level"=2, "Descriptive Name"="Clear Errors", "Class Only"=FALSE, "Data Type"=4, "Access"=1, "Identifier"="RSZVL_ATTR_SYST_ERR_CLEAR", "Range Table"="", "Command"="SYST:ERR:CLE:ALL", "Read Callback"="", "Write Callback"="", "Range Callback"="", "Check Callback"="", "Rngtable Callback"="", "Coerce Callback"="", "User Callback"="", "Supported Models"="", "Instrument Options"="", "Repeated Capabilities"="", "Restricted Repeated Capabilities"="", "Help"="This attribute deletes all entries in the table SYSTEM MESSAGES.\n\nAvailable Repeated Capabilities:\nNone\n\nRemote-control command(s):\nSYSTem:ERRor:CLEar:ALL", "Flags"={"OPC Wait"=FALSE, "Dont check status"=FALSE, "*WAI"=FALSE}, "Check Status Callback"=""}, {"Level"=2, "Descriptive Name"="System Preset", "Class Only"=FALSE, "Data Type"=4, "Access"=1, "Identifier"="RSZVL_ATTR_SYST_PRESET", "Range Table"="", "Command"="SYST:PRES", "Read 
